vi "Check is timestamp.vi"(8 "error in (no error)":errorcluster, 11 "MessagePack.lvlib:MsgPackTimestamp.lvclass":refnum<class "MsgPackTimestamp.lvclass">) -> (0 "error out":errorcluster, 2 "Valid?":bool, 3 "MessagePack.lvlib:MsgPackTimestamp.lvclass 2":refnum<class "MsgPackTimestamp.lvclass">)   [LabVIEW 2020, in "MessagePack.lvlib" / "MsgPackTimestamp.lvclass"]
uses:
  MsgPackTimestamp.lvclass
  MsgPackTimestamp.lvclass/MsgPackTimestamp.ctl
  MsgPackExt/MsgPackExt.lvclass
  C:/local/wamplv/MessagePack/MsgPackExt/MsgPackExt.lvclass
  C:/local/wamplv/MessagePack/IMessagePackObject/IMessagePackObject.lvclass
  C:/local/wamplv/MessagePack/MsgPackTimestamp/MsgPackTimestamp.lvclass
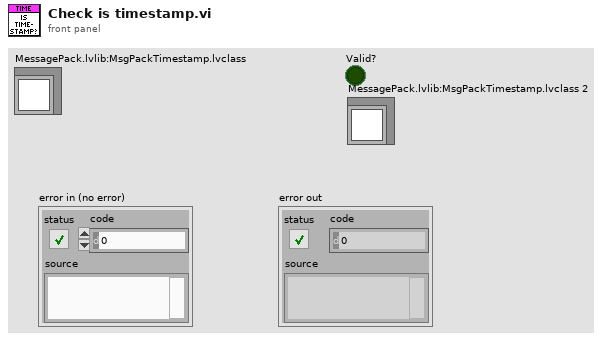
[diagram p1: front panel]
types:
  T1 = typedef "MessagePack.lvlib/MsgPack Object Types.ctl" = enum16{"UNSUPPORTED", "POSINT", "NEGINT", "FIXMAP", "FIXARRAY", "FIXSTR", "NIL", "FALSE", "TRUE", "BIN8", "BIN16", "BIN32", "EXT8", "EXT16", "EXT32", "FLOAT32", "FLOAT64", "UINT8", "UINT16", "UINT32", "UINT64", "INT8", "INT16", "INT32", "INT64", "FIXEXT1", "FIXEXT2", "FIXEXT4", "FIXEXT8", "FIXEXT16", "STR8", "STR16", "STR32", "ARRAY16", "ARRAY32", "MAP16", "MAP32"}
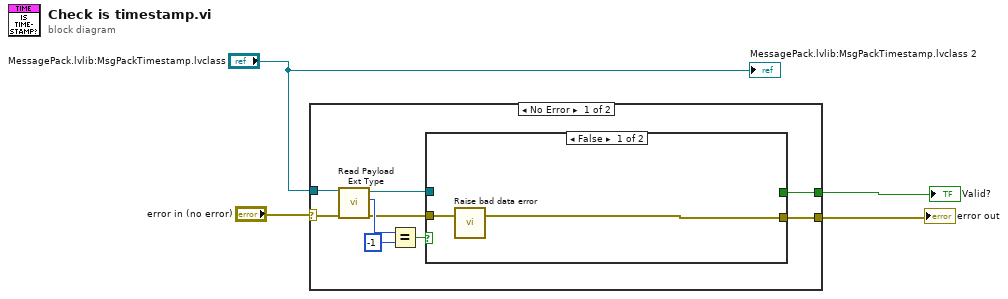
[diagram p0: block diagram]
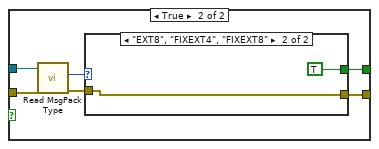
[diagram p2: hidden frame]
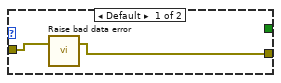
[diagram p3: hidden frame]
diagram:
  n1 = case shown="No Error" "error in (no error)" {
    selector: "error in (no error)" -> [w13 w26]
    tunnel: [w7 w26] -> w4
    tunnel: "MessagePack.lvlib:MsgPackTimestamp.lvclass" -> [w12 _]
    tunnel: [w5 _] -> w2
    frame No Error {
      n2 = call "Read Payload Ext Type.vi"("error in (no error)"=w13, "MsgPackExt in"=w12) -> ("error out"=w8:errorcluster, "Payload Ext Type"=w11:i8, "MsgPackExt out"=w6:refnum<class "MsgPackTimestamp.lvclass">)  [unwired: 7 in]
      n3 = Equal?(x=w11, y=i8 -1) -> (x = y?=w9:bool)
      n4 = case shown="False" w9 {
        tunnel: w8 -> [w15 w21]
        tunnel: [w14 w17] -> w7
        tunnel: w6 -> [_ w20]
        tunnel: [_ w16] -> w5
        frame False {
          n5 = call "Raise bad data error.vi"("error in (no error)"=w15) -> ("error out"=w14:errorcluster)  [unwired: 2 in]
        }
        frame True {
          n6 = call "Read MsgPack Type.vi"("error in (no error)"=w21, "MsgPackExt in"=w20) -> ("error out"=w18:errorcluster, "MsgPack Object Type"=w19:T1)  [unwired: 7 in, 1 out]
          n7 = case shown="\"EXT8\", \"FIXEXT4\", \"FIXEXT8\"" w19 {
            tunnel: w18 -> [w23 w25]
            tunnel: [w22 w25] -> w17
            tunnel: [_ TRUE] -> w16
            frame Default {
              n8 = call "Raise bad data error.vi"("error in (no error)"=w23) -> ("error out"=w22:errorcluster)  [unwired: 2 in]
            }
            frame "EXT8", "FIXEXT4", "FIXEXT8" {
            }
          }
        }
      }
    }
    frame Error {
    }
  }
  "error out" <- w4
  "Valid?" <- w2
  "MessagePack.lvlib:MsgPackTimestamp.lvclass 2" <- "MessagePack.lvlib:MsgPackTimestamp.lvclass"
